vi "Initialize Caves.vi"(11 "array type (2D Dbl)":string[][](array[string])) -> (2 "Array":T1[](array[typedef]), 3 "array":string[][](array[string]))   [LabVIEW 2019, in "Day 12.lvlib"]
uses:
  Day 12.lvlib
  Controls/Cave.ctl
  Controls/Cave Type.ctl
  43343be5-61f0-47a1-bb9c-4ba9e4b56087.vi
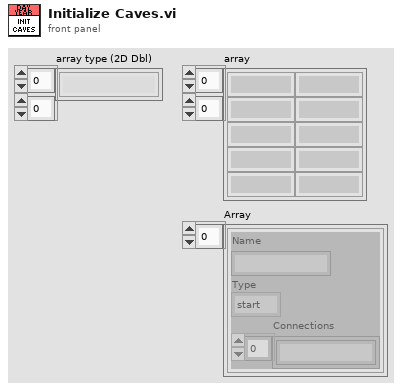
[diagram p1: front panel]
types:
  T1 = typedef "Day 12.lvlib/Cave.ctl" = cluster{"Name":string, "Type":T2, "Connections":string[]}
  T2 = typedef "Day 12.lvlib/Cave Type.ctl" = enum16{"start", "end", "small", "big"}
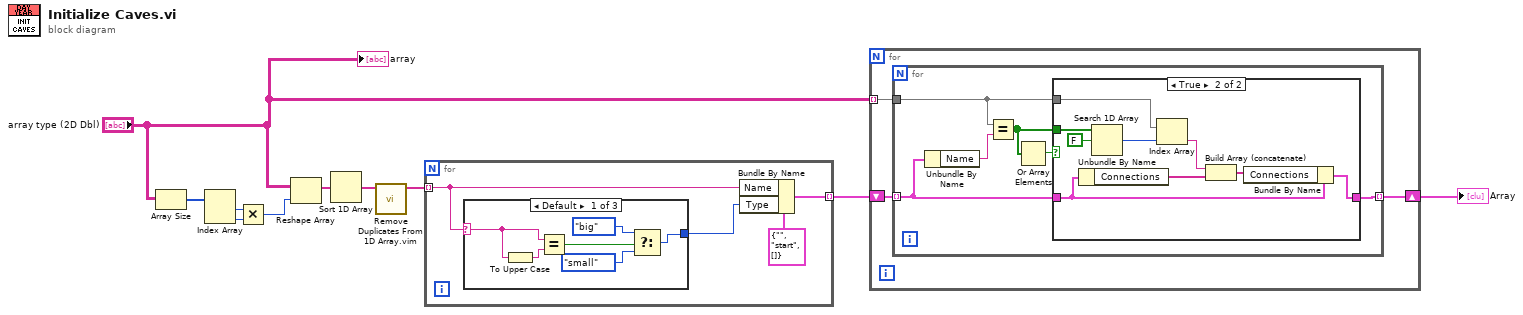
[diagram p0: block diagram]
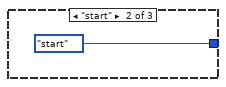
[diagram p3: hidden frame]
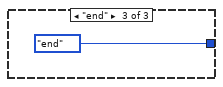
[diagram p4: hidden frame]
diagram:
  n1 = Array Size(array="array type (2D Dbl)") -> (size(s)=w1:i32[])
  n2 = Index Array(array=w1) -> (element #1=w3:i32, element #2=w2:i32)  [unwired: 2 in]
  n3 = Multiply(x=w3, y=w2) -> (x*y=w4:i32)
  n4 = Reshape Array("array type (2D Dbl)", w4) -> (w5:string[])
  n5 = Sort 1D Array(array=w5) -> (sorted array=w6:string[])
  n6 = call "Remove Duplicates From 1D Array.vim"("array"=w6) -> ("array with duplicates removed"=w7:string[])  [unwired: 10 in]
  n7 = for {
    tunnel: w7 -> [w13] mode=indexing
    tunnel: [w11] -> w9 mode=indexing
    n8 = case shown="Default" w13 {
      selector: w13 -> [w20 _ _]
      tunnel: [w15 Cave_Type."start" ("Type") Cave_Type."end" ("Type")] -> w12
      frame Default {
        n9 = To Upper Case(1:w20) -> (0:w19:string)
        n10 = Equal?(x=w20, y=w19) -> (x = y?=w18:bool)
        n11 = Select(t=Cave_Type."big" ("Type"), s=w18, f=Cave_Type."small" ("Type")) -> (s? t:f=w15:T2)
      }
      frame "start" {
      }
      frame "end" {
      }
    }
    n12 = Bundle By Name(cluster=T1 {"Name"="", "Type"=enum."start", "Connections"=[]} ("Cave"), "Name"=w13, "Type"=w12) -> (w11:T1)
  }
  n13 = for {
    tunnel: "array type (2D Dbl)" -> [w24] mode=indexing
    shift-right: [w23] -> w10
    shift-left: w9 -> [w25]
    n14 = for {
      tunnel: w25 -> [w31] mode=indexing
      tunnel: w24 -> [w27]
      tunnel: [w28] -> w23 mode=indexing
      n15 = Unbundle By Name(w31) -> ("Name"=w30:string)
      n16 = Equal?(x=w27, y=w30) -> (x = y?=w26:bool[])
      n17 = Or Array Elements(Boolean array=w26) -> (logical OR=w29:bool)
      n18 = case shown="True" w29 {
        tunnel: w31 -> [w32 w40]
        tunnel: [w32 w41] -> w28
        tunnel: w27 -> [_ w37]
        tunnel: w26 -> [_ w39]
        frame False {
        }
        frame True {
          n19 = Unbundle By Name(w40) -> ("Connections"=w34:string[])
          n20 = Search 1D Array(1D array=w39, element=FALSE) -> (index of element=w36:i32)  [unwired: 1 in]
          n21 = Index Array(array=w37, index=w36) -> (element=w35:string)
          n22 = Build Array (concatenate)(w35, w34) -> (w33:string[])
          n23 = Bundle By Name(cluster=w40, "Connections"=w33) -> (w41:T1)
        }
      }
    }
  }
  "Array" <- w10
  "array" <- "array type (2D Dbl)"
